vi "UEvent_MEASURE_FULL_PROCESS_START.vi"(0 "Refnum in":refnum<k21>, 5 "Range - Shunts":T1, 7 "Ext PW Vol Monitor":bool=TRUE, 9 "USB":tag, 11 "Internal/external Power":bool=TRUE, 12 "Vout  - Vbat profile":enum16{"3.8VDC", "2.9VDC", "By Pass", "4.0VDC"}(ring), 13 "Sample rate":u32=20000) -> (1 "DevSerialNum":u32, 3 "Power ON/OFF":bool, 4 "Refnum out":refnum<k21>, 6 "Battery_Voltage":dbl, 10 "DUT_Voltage":dbl, 14 "Measure indicator":bool=TRUE, 15 "error out":errorcluster)   [LabVIEW 2017]
uses:
  Range_Shunt_selector.ctl
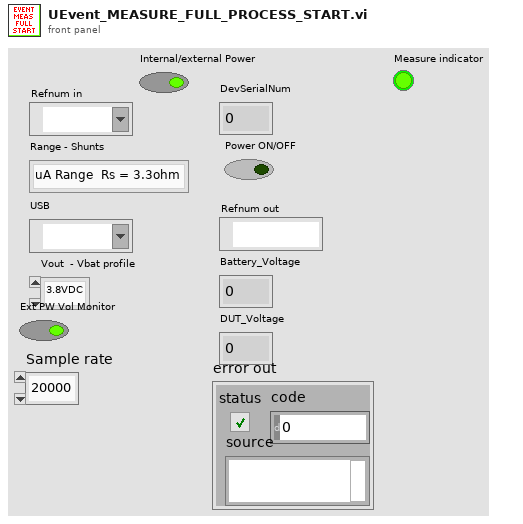
[diagram p1: front panel]
types:
  T1 = typedef "Range_Shunt_selector.ctl" = enum16{"uA Range  Rs = 3.3ohm", "mA Range Rs = 3.3ohm", "mA Range Rs = 1ohm", "mA Range Rs = 1ohm - X2"}
  T2 = enum16{"Internal PW Source", "External PW Source"}
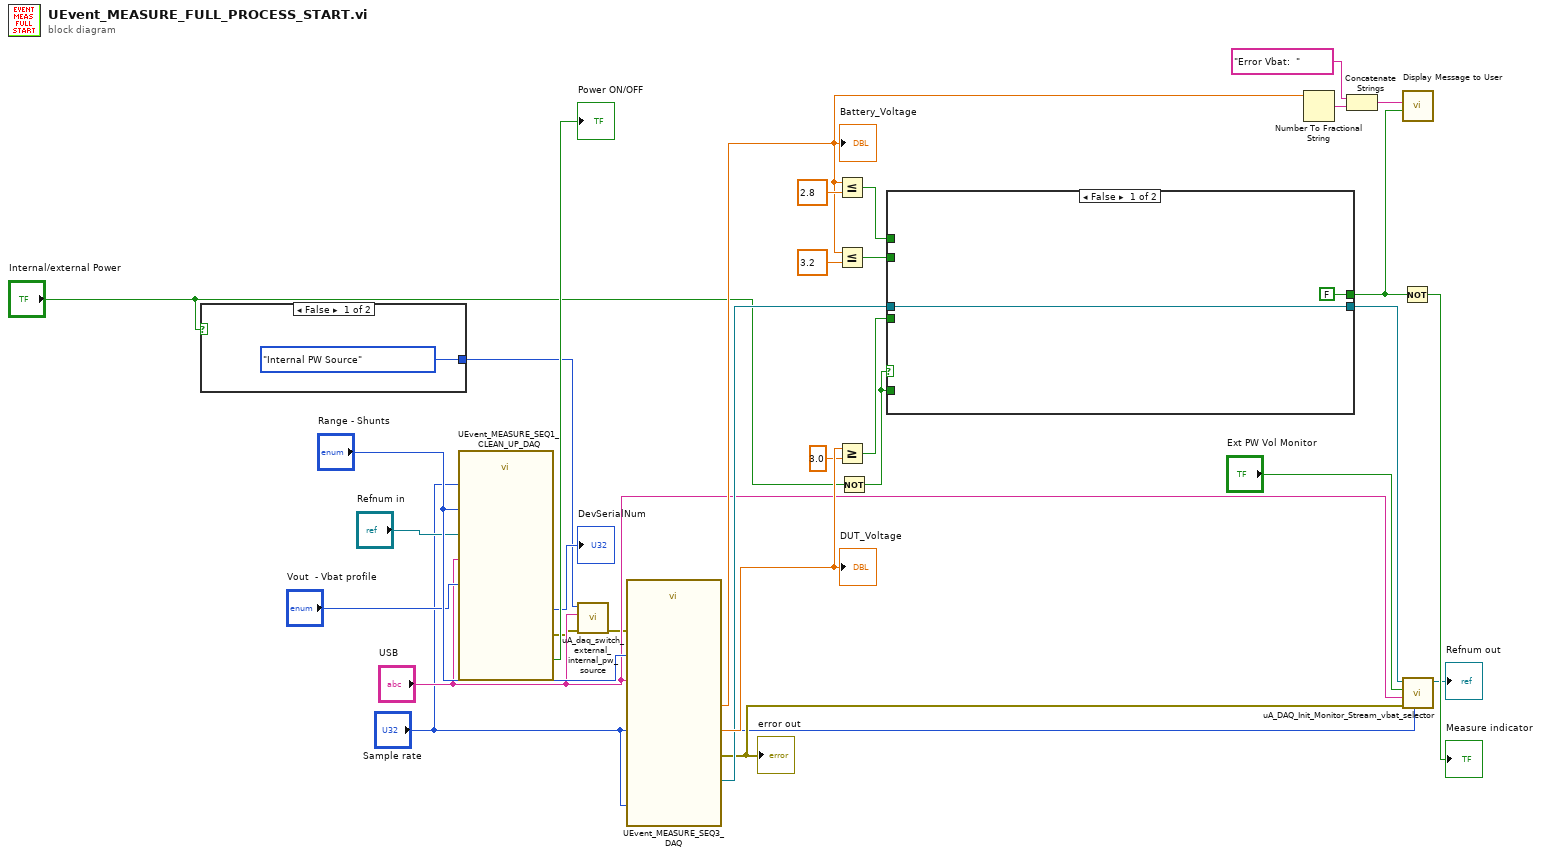
[diagram p0: block diagram]
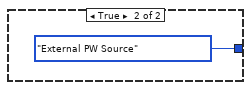
[diagram p2: hidden frame]
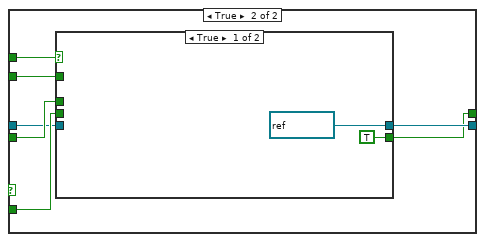
[diagram p3: hidden frame]
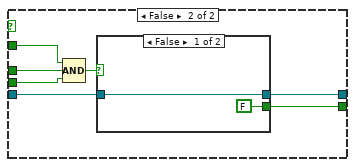
[diagram p4: hidden frame]
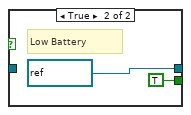
[diagram p5: hidden frame]
diagram:
  n1 = case shown="False" "Internal/external Power" {
    tunnel: [T2."Internal PW Source" ("Ex/Int PW") T2."External PW Source" ("Ex/Int PW")] -> w5
    frame False {
    }
    frame True {
    }
  }
  n2 = call "UEvent_MEASURE_SEQ1_CLEAN_UP_DAQ.vi"("USB  in"="USB", "rate"="Sample rate", "Vout  - Vbat profile"="Vout  - Vbat profile", "Range - Shunts in"="Range - Shunts", "TASK IN"="Refnum in") -> ("error out"=w2:errorcluster, "DevSerialNum"=→"DevSerialNum":u32, "Power ON/OFF"=→"Power ON/OFF":bool)  [unwired: 4 in]
  n3 = call "uA_daq_switch_external_internal_pw_source.vi"("error in"=w2, "USB DAQ"="USB", "Ex/Int PW"=w5) -> ("error out"=w3:errorcluster)  [unwired: 8 in]
  n4 = call "UEvent_MEASURE_SEQ3_DAQ.vi"("rate"="Sample rate", "error in (no error)"=w3, "USB in"="USB", "Range - Shunts"="Range - Shunts") -> ("error out"=w9:errorcluster, "DUT_Voltage"=w24:dbl, "Battery_Voltage"=w18:dbl, "Refnum out"=w20:refnum<k21>)  [unwired: 4 in]
  "DUT_Voltage" <- w24
  "Battery_Voltage" <- w18
  "error out" <- w9
  n5 = Less Or Equal?(x=w18, y=2.8) -> (x <= y?=w13:bool)
  n6 = Less Or Equal?(x=w18, y=3.2) -> (x <= y?=w22:bool)
  n7 = Greater Or Equal?(x=w24, y=3.0) -> (x >= y?=w21:bool)
  n8 = Not(x="Internal/external Power") -> (.not. x?=w12:bool)
  n9 = case shown="False" w12 {
    tunnel: w22 -> [_ w41]
    tunnel: w21 -> [_ w40]
    tunnel: w12 -> [_ w39]
    tunnel: w20 -> [w34 w38]
    tunnel: [w34 w37] -> w8
    tunnel: [FALSE ("Enable") w36] -> w14
    tunnel: w13 -> [_ w35]
    frame False {
    }
    frame True {
      n10 = case shown="True" w35 {
        tunnel: w41 -> [_ w50]
        tunnel: w40 -> [_ w49]
        tunnel: w39 -> [_ w47]
        tunnel: w38 -> [_ w46]
        tunnel: [refnum<k21> "Stop" ("y") w45] -> w37
        tunnel: [TRUE ("Enable") w44] -> w36
        frame True {
        }
        frame False {
          n11 = Compound Arithmetic op=AND(w50, w49, w47) -> (w48:bool)
          n12 = case shown="False" w48 {
            tunnel: w46 -> [w52 _]
            tunnel: [w52 refnum<k21> "Stop" ("y")] -> w45
            tunnel: [FALSE ("Enable") TRUE ("Enable")] -> w44
            frame False {
            }
            frame True {
              # "Low Battery"
            }
          }
        }
      }
    }
  }
  n13 = Number To Fractional String(number=w18) -> (F-format string=w17:string)  [unwired: 3 in]
  n14 = Concatenate Strings("Error Vbat:  " ("string"), w17) -> (w15:string)
  n15 = Not(x=w14) -> (.not. x?=→"Measure indicator":bool)
  n16 = call "Display Message to User"("Enable"=w14, "Message"=w15) -> ()  [unwired: 8 in, 2 out]
  n17 = call "uA_DAQ_Init_Monitor_Stream_vbat_selector.vi"("Sample rate"="Sample rate", "error in (no error)"=w9, "USB"="USB", "Ext PW Vol Monitor"="Ext PW Vol Monitor", "Refnum in"=w8) -> ("Refnum out"=→"Refnum out":refnum<k21>)  [unwired: 5 in, 1 out]
